vi "I_Sense_v3.vi"(8 "error in":errorcluster, 9 "Cycles":i32=10, 10 "Test Freq":enum16{"10Hz", "100Hz", "1kHz", "5kHz"}(ring), 11 "Choose Test":T1(ring)) -> (0 "error out":errorcluster, 3 "Result":dbl[](array[numeric]))   [LabVIEW 2021]
uses:
  <vilib>/DAQmx/write.llb/DAQmx Write (Analog 1D Wfm NChan NSamp).vi
  <vilib>/DAQmx/read.llb/DAQmx Read (Analog 1D Wfm NChan NSamp).vi
  <vilib>/DAQmx/create/channels.llb/DAQmx Create Channel (AO-Voltage-Basic).vi
  <vilib>/DAQmx/configure/timing.llb/DAQmx Timing (Sample Clock).vi
  <vilib>/measure/mascope.llb/Amplitude and Levels N chan.vi
  <vilib>/DAQmx/miscellaneous.llb/DAQmx Fill In Error Info.vi
  <vilib>/DAQmx/create/channels.llb/DAQmx Create Channel (AI-Voltage-Basic).vi
  <vilib>/measure/madcrms.llb/Basic Averaged DC-RMS for N Chan.vi
  <resource>/objmgr/daqmx.rc
  <vilib>/measure/NI_MABase.lvlib
  <vilib>/measure/NI_MAPro.lvlib
panel:
  out "DC values":dbl[](array[numeric]) format="%.2p"
  out "Gains":dbl[](array[numeric])
  out "Amplitude Out":dbl[](array[numeric]) format="%.2p"
  out "High Out":dbl[](array[numeric]) format="%.2p"
  out "Low Out":dbl[](array[numeric]) format="%.2p"
  out "Amplitude In":dbl[](array[numeric]) format="%.2p"
  out "Low In":dbl[](array[numeric]) format="%.2p"
  out "High In":dbl[](array[numeric]) format="%.2p"
  in  "Sample Mode":i32(ring)=10123 items=["Finite Samples"=10178, "Continuous Samples"=10123, "Hardware Timed Single Point"=12522]
  out "Output Waveform":waveform(dbl)[](graph)=[{"t0"=timestamp(0 s since 1904-01-01), "dt"=0.001, "Y"=[]}]
  out "Input Waveform":waveform(dbl)[](graph)=[{"t0"=timestamp(0 s since 1904-01-01), "dt"=0.001, "Y"=[]}]
  in  "Sample Clock Source":tag="OnboardClock"
  out "Actual Sample Rate":dbl=1000.0 format="%0.2f"
  # "ISENSE_C+"
  # "ISENSE_C-"
  # "ISENSE_C+"
  # "ISENSE_C-"
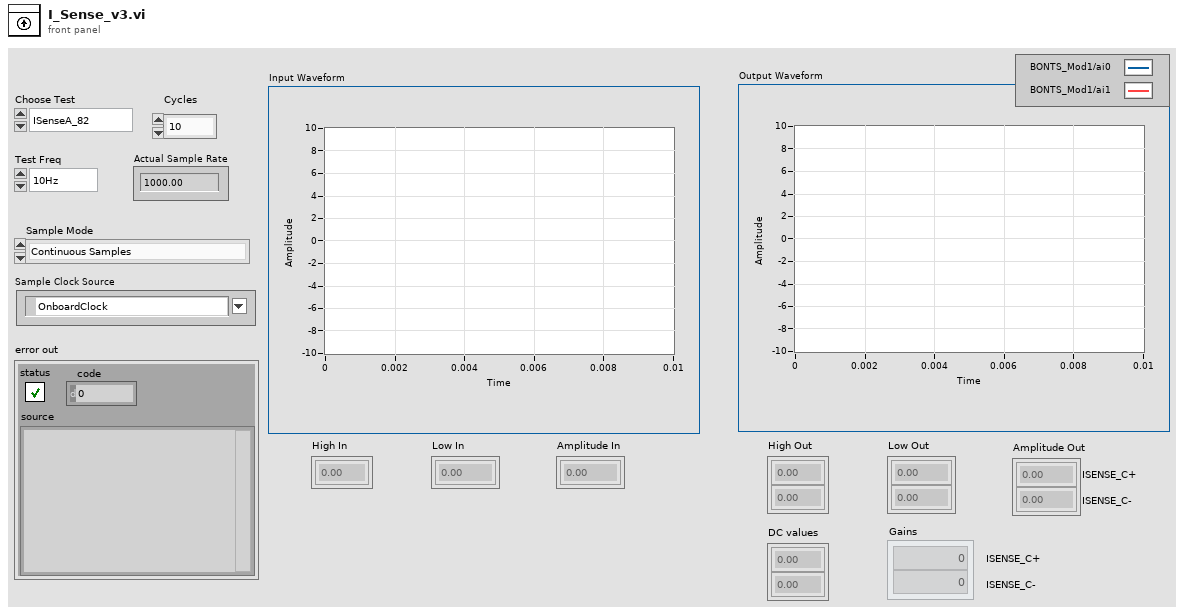
[diagram p1: front panel]
types:
  T1 = enum16{"ISenseA_82", "ISenseB_82", "ISenseC_82", "ISenseC_92", "ISenseA_93", "ISenseC_93"}
  T2 = cluster{"Waveform Type":u16, "Amplitude":dbl, "Frequency":dbl}[]
  T3 = cluster{"Waveform Type":u16, "Amplitude":dbl, "Frequency":dbl}
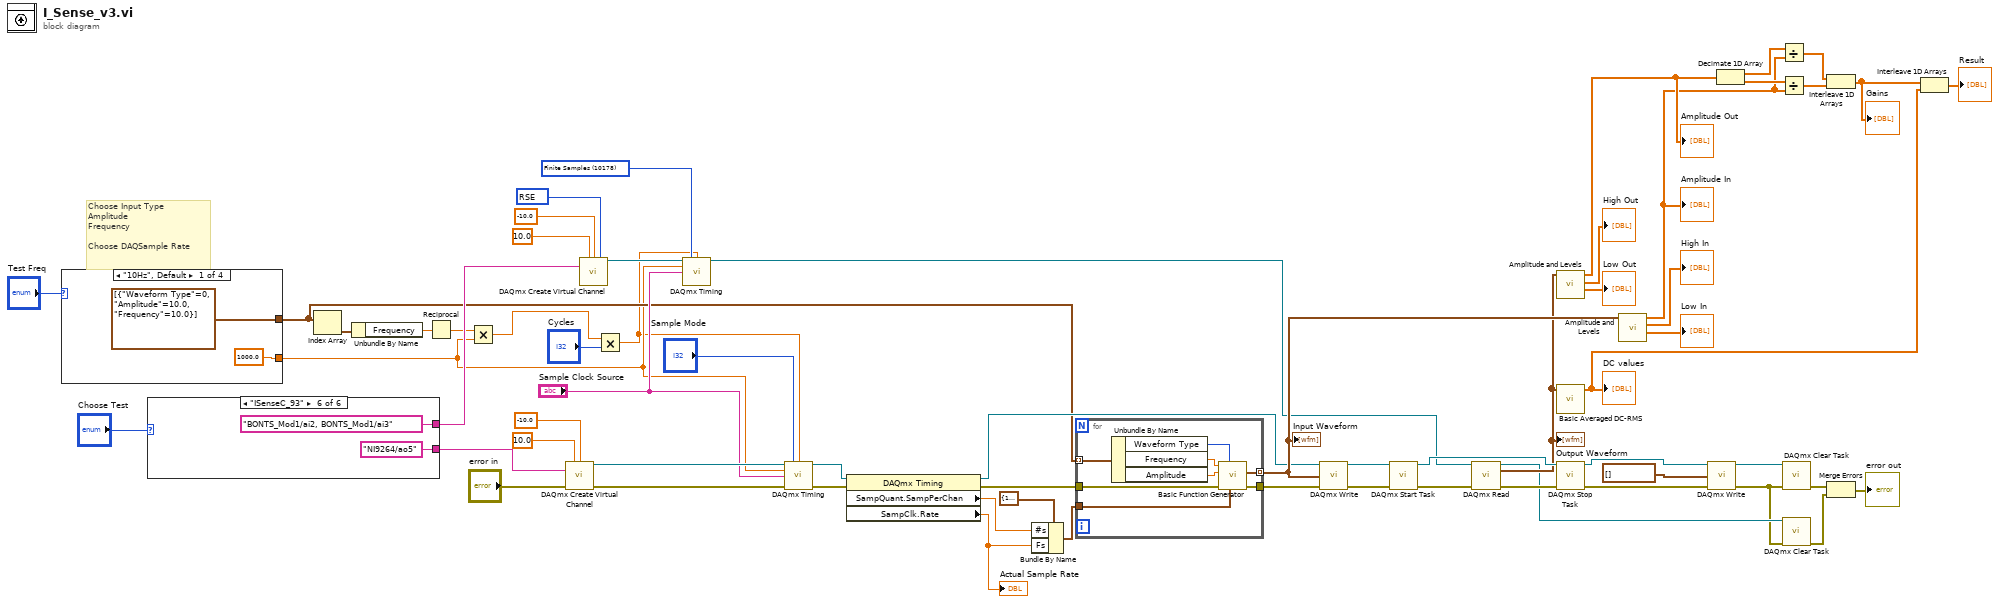
[diagram p0: block diagram]
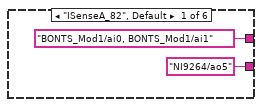
[diagram p2: hidden frame]
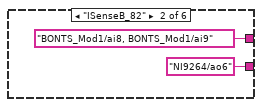
[diagram p3: hidden frame]
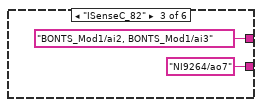
[diagram p4: hidden frame]
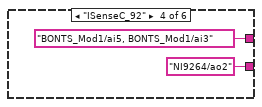
[diagram p5: hidden frame]
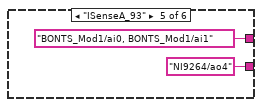
[diagram p6: hidden frame]
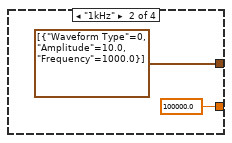
[diagram p7: hidden frame]
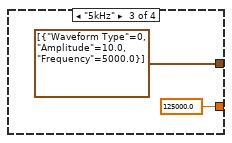
[diagram p8: hidden frame]
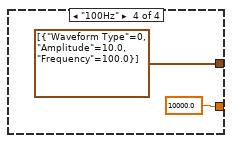
[diagram p9: hidden frame]
diagram:
  w1 = 10083 items=["Default"=-1, "RSE"=10083, "NRSE"=10078, "Differential"=10106, "Pseudodifferential"=12529] ("input terminal configuration")
  w18 = 10178 items=["Finite Samples"=10178, "Continuous Samples"=10123, "Hardware Timed Single Point"=12522] ("sample mode")
  # "Choose Input Type\nAmplitude \nFrequency\n\nChoose DAQSample Rate"
  n1 = case shown="\"10Hz\", Default" "Test Freq" {
    tunnel: [1000.0 ("Sample Rate") 100000.0 ("Sample Rate") 125000.0 ("Sample Rate") 10000.0 ("Sample Rate")] -> w6
    tunnel: [T2 [{"Waveform Type"=0, "Amplitude"=10.0, "Frequency"=10.0}] ("Output Array") T2 [{"Waveform Type"=0, "Amplitude"=10.0, "Frequency"=1000.0}] ("Output Array") T2 [{"Waveform Type"=0, "Amplitude"=10.0, "Frequency"=5000.0}] ("Output Array") T2 [{"Waveform Type"=0, "Amplitude"=10.0, "Frequency"=100.0}] ("Output Array")] -> w10
    frame "10Hz", Default {
    }
    frame "1kHz" {
    }
    frame "5kHz" {
    }
    frame "100Hz" {
    }
  }
  n2 = case shown="\"ISenseC_93\"" "Choose Test" {
    tunnel: ["NI9264/ao5" ("Write Channel(s)") "NI9264/ao6" ("Write Channel(s)") "NI9264/ao7" ("Write Channel(s)") "NI9264/ao2" ("Write Channel(s)") "NI9264/ao4" ("Write Channel(s)") "NI9264/ao5" ("Write Channel(s)")] -> w28
    tunnel: ["BONTS_Mod1/ai0, BONTS_Mod1/ai1" ("Read Channel(s)") "BONTS_Mod1/ai8, BONTS_Mod1/ai9" ("Read Channel(s)") "BONTS_Mod1/ai2, BONTS_Mod1/ai3" ("Read Channel(s)") "BONTS_Mod1/ai5, BONTS_Mod1/ai3" ("Read Channel(s)") "BONTS_Mod1/ai0, BONTS_Mod1/ai1" ("Read Channel(s)") "BONTS_Mod1/ai2, BONTS_Mod1/ai3" ("Read Channel(s)")] -> w11
    frame "ISenseA_82", Default {
    }
    frame "ISenseB_82" {
    }
    frame "ISenseC_82" {
    }
    frame "ISenseC_92" {
    }
    frame "ISenseA_93" {
    }
    frame "ISenseC_93" {
    }
  }
  n3 = Index Array(array=w10) -> (element=w9:T3)  [unwired: 1 in]
  n4 = Unbundle By Name(w9) -> ("Frequency"=w8:dbl)
  n5 = Reciprocal(x=w8) -> (1/x=w7:dbl)
  n6 = Multiply(x=w7, y=w6) -> (x*y=w5:dbl)
  n7 = call-poly <vilib>:"DAQmx Create Virtual Channel.vi"("maximum value"=10.0, "minimum value"=-10.0, "physical channels"=w28, "error in"="error in") -> ("task out"=w60:refnum<k21>, "error out"=w61:errorcluster)  [unwired: 10 in]
  n8 = call-poly <vilib>:"DAQmx Create Virtual Channel.vi"("maximum value"=10.0, "minimum value"=-10.0, "input terminal configuration"=w1, "physical channels"=w11) -> ("task out"=w22:refnum<k21>)  [unwired: 10 in, 1 out]
  n9 = Multiply(x=w5, y="Cycles") -> (x*y=w4:dbl)
  n10 = call-poly <vilib>:"DAQmx Timing.vi"("task/channels in"=w22, "sample mode"=w18, "samples per channel"=w4, "rate"=w6, "source"="Sample Clock Source") -> ("task out"=w21:refnum<k21>)  [unwired: 9 in, 1 out]
  n11 = call-poly <vilib>:"DAQmx Timing.vi"("task/channels in"=w60, "sample mode"="Sample Mode", "samples per channel"=w4, "rate"=w6, "source"="Sample Clock Source", "error in"=w61) -> ("task out"=w30:refnum<k21>, "error out"=w63:errorcluster)  [unwired: 8 in]
  n12 = property class="DAQmx Timing"(reference=w30, error in=w63) -> (reference out=w27:refnum<k21>, error out=w51:errorcluster, "SampQuant.SampPerChan"=w54:dbl, "SampClk.Rate"=w53:dbl)
  "Actual Sample Rate" <- w53
  n13 = Bundle By Name(cluster=cluster{"Fs":dbl, "#s":dbl} {"Fs"=1000.0, "#s"=1000.0} ("sampling info"), "#s"=w54, "Fs"=w53) -> (w58:cluster{"Fs":dbl, "#s":dbl})
  n14 = for {
    tunnel: w51 -> [w91]
    tunnel: w58 -> [w90]
    tunnel: [w89] -> w55
    tunnel: w10 -> [w88] mode=indexing
    tunnel: [w84] -> w46 mode=indexing
    n15 = Unbundle By Name(w88) -> ("Waveform Type"=w87:u16, "Frequency"=w86:dbl, "Amplitude"=w85:dbl)
    n16 = call <vilib>:"Basic Function Generator.vi"("sampling info"=w90, "signal type"=w87, "error in (no error)"=w91, "amplitude"=w85, "frequency"=w86) -> ("error out"=w89:errorcluster, "signal out"=w84:waveform(dbl))  [unwired: 4 in, 1 out]
  }
  "Input Waveform" <- w46
  n17 = call-poly <vilib>:"DAQmx Write.vi"("task/channels in"=w27, "data"=w46, "error in"=w55) -> ("task out"=w57:refnum<k21>, "error out"=w56:errorcluster)  [unwired: 10 in, 1 out]
  n18 = call <vilib>:"DAQmx Start Task.vi"("task/channels in"=w57, "error in"=w56) -> ("task out"=w52:refnum<k21>, "error out"=w50:errorcluster)  [unwired: 12 in]
  n19 = call-poly <vilib>:"DAQmx Read.vi"("task/channels in"=w21, "error in"=w50) -> ("task out"=w20:refnum<k21>, "data"=w34:waveform(dbl)[], "error out"=w49:errorcluster)  [unwired: 11 in]
  "Output Waveform" <- w34
  n20 = call-poly <vilib>:"Amplitude and Levels.vi"("signal(s) in"=w34) -> ("low state level"=→"Low Out":dbl[], "high state level"=→"High Out":dbl[], "amplitude"=w40:dbl[])  [unwired: 7 in, 1 out]
  "Amplitude Out" <- w40
  n21 = call-poly <vilib>:"Basic Averaged DC-RMS.vi"("signals in"=w34) -> ("DC values"=w32:dbl[])  [unwired: 7 in, 3 out]
  "DC values" <- w32
  n22 = call <vilib>:"DAQmx Stop Task.vi"("task/channels in"=w52, "error in"=w49) -> ("task out"=w25:refnum<k21>, "error out"=w26:errorcluster)  [unwired: 12 in]
  n23 = call-poly <vilib>:"Amplitude and Levels.vi"("signal(s) in"=w46) -> ("low state level"=→"Low In":dbl[], "high state level"=→"High In":dbl[], "amplitude"=w37:dbl[])  [unwired: 7 in, 1 out]
  "Amplitude In" <- w37
  n24 = call-poly <vilib>:"DAQmx Write.vi"("task/channels in"=w25, "data"=waveform(dbl)[] [], "error in"=w26) -> ("task out"=w24:refnum<k21>, "error out"=w19:errorcluster)  [unwired: 10 in, 1 out]
  n25 = Decimate 1D Array(w40) -> (w39:dbl[], w38:dbl[])
  n26 = Divide(x=w39, y=w37) -> (x/y=w36:dbl[])
  n27 = Divide(x=w38, y=w37) -> (x/y=w35:dbl[])
  n28 = call <vilib>:"DAQmx Clear Task.vi"("task in"=w24, "error in"=w19) -> ("error out"=w16:errorcluster)  [unwired: 13 in]
  n29 = call <vilib>:"DAQmx Clear Task.vi"("task in"=w20, "error in"=w19) -> ("error out"=w15:errorcluster)  [unwired: 13 in]
  n30 = Interleave 1D Arrays(w36, w35) -> (w33:dbl[])
  "Gains" <- w33
  n31 = Merge Errors(w16, w15) -> (→"error out":errorcluster)
  n32 = Interleave 1D Arrays(w33, w32) -> (→"Result":dbl[])
